vi "ContextHelp_LeavingDialog.vi"(5 "error in (no error)":errorcluster) -> (19 "error out":errorcluster)   [LabVIEW 2016]
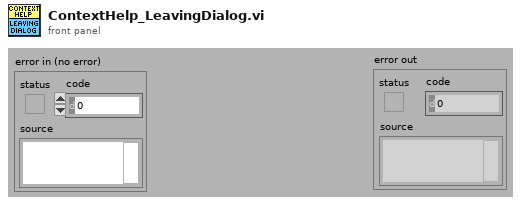
[diagram p1: front panel]
types:
  T1 = enum16{"SetPopUpEventTask", "GetStatus", "SetOpenState", "SetDialogCaller", "SetToolHelp"}
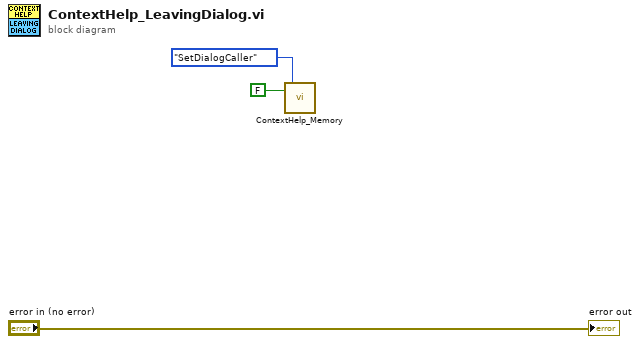
[diagram p0: block diagram]
diagram:
  n1 = call <resource>:"ContextHelp_Memory.vi"("State"=FALSE, "Actio(GetStatus)n"=T1."SetDialogCaller") -> ()  [unwired: 2 in, 16 out]
  "error out" <- "error in (no error)"
